vi "Correction_Factor.vi"(9 "Z in":dbl, 10 "Y in":dbl, 11 "X in":dbl) -> (1 "Z out":dbl, 2 "Y out":dbl, 3 "X out":dbl)   [LabVIEW 2011]
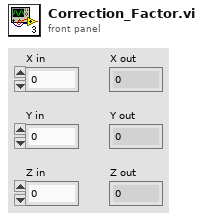
[diagram p1: front panel]
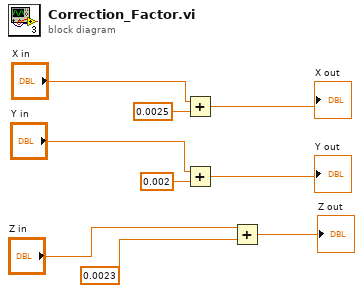
[diagram p0: block diagram]
diagram:
  n1 = Add(x="X in", y=0.0025) -> (x+y=→"X out":dbl)
  n2 = Add(x="Y in", y=0.002) -> (x+y=→"Y out":dbl)
  n3 = Add(x="Z in", y=0.0023) -> (x+y=→"Z out":dbl)
